vi "TEST.vi"() -> ()   [LabVIEW 2018, in "Config Parser BML.lvlib" / "Config Parser BML.lvclass"]
uses:
  Config Parser BML.lvclass
  Ctls/FRM Data - BML.ctl
  Ctls/OM - BML.ctl
  Ctls/Burst Length.ctl
  Ctls/RW Options.ctl
  Interfaces/File Parser Interface.lvlibp/Ctls/Protocol Type.ctl
  Interfaces/File Parser Interface.lvlibp/Interfaces/File Parser Interface/File Parser Interface.lvclass
  Interfaces/File Parser Interface.lvlibp
  C:/P4 Workspace/PC Client/Solutions/5g_eap/trunk/1.0/HiSi5GmmWave/Pattern_Gen_Tool/Interfaces/File Parser Interface.lvlibp/Interfaces/File Parser Interface/File Parser Interface.lvclass
panel:
  out "Array":T1[](array[typedef]) {"ChipID" format="%x"; "Start_Addr" format="%x"; "Data" format="%x"}
  out "error out":errorcluster
  in  "Config File":path
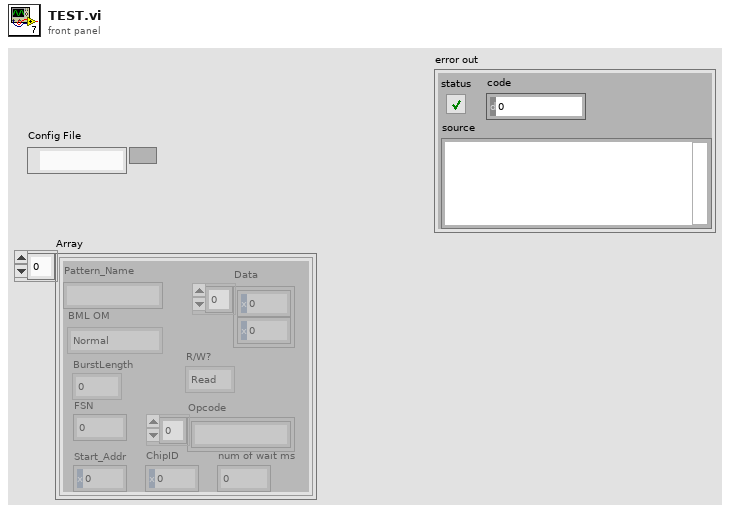
[diagram p1: front panel]
types:
  T1 = typedef "FRM Data - BML.ctl" = cluster{"Pattern_Name":string, "Data":u8[], "Start_Addr":u16, "ChipID":u8, "num of wait ms":i8, "Opcode":string[], "BML OM":T2, "BurstLength":T3, "FSN":u8, "R/W?":T4}
  T2 = typedef "OM - BML.ctl" = enum16{"Normal", "ImmeEffect", "InitSlaveID", "LoadData"}
  T3 = typedef "Burst Length.ctl" = enum8{"0", "2", "3", "4", "5", "8", "16", "32"}
  T4 = typedef "RW Options.ctl" = enum16{"Read", "Write", "R/W"}
  T5 = typedef "File Parser Interface.lvlibp/Protocol Type.ctl" = enum16{"BML_LS", "BML_HS", "SPI_3W", "SPI_4W"}
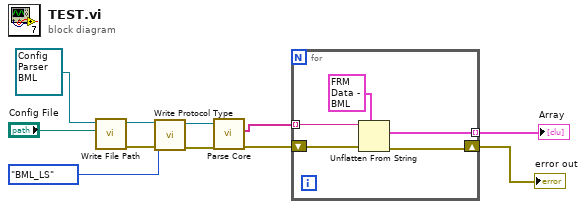
[diagram p0: block diagram]
diagram:
  n1 = call "Write File Path.vi"("File Path"="Config File", "File Parser Interface in"=refnum<class "Config Parser BML.lvclass"> refnum ("Config Parser BML.lvlib:Config Parser BML.lvclass")) -> ("error out"=w3:errorcluster, "File Parser Interface out"=w5:refnum<class "Config Parser BML.lvclass">)  [unwired: 8 in]
  n2 = call "Write Protocol Type.vi"("error in (no error)"=w3, "Protocol Type"=Protocol_Type."BML_LS", "File Parser Interface in"=w5) -> ("error out"=w2:errorcluster, "File Parser Interface out"=w4:refnum<class "Config Parser BML.lvclass">)  [unwired: 7 in]
  n3 = call-dynamic "Parse Core.vi"("error in (no error)"=w2, "Config Parser BML in"=w4) -> ("error out"=w7:errorcluster, "Config Array"=w6:string[])  [unwired: 7 in, 1 out]
  n4 = for {
    tunnel: [w15] -> w10 mode=indexing
    shift-right: [w13] -> w11
    shift-left: w7 -> [w14]
    tunnel: w6 -> [w12] mode=indexing
    n5 = Unflatten From String(type=T1 {"Pattern_Name"="", "Data"=[], "Start_Addr"=0, "ChipID"=1, "num of wait ms"=0, "Opcode"=[], "BML OM"=enum."Normal", "BurstLength"=enum."0", "FSN"=0, "R/W?"=enum."Read"} ("Frame Data"), binary string=w12, error in (no error)=w14) -> (value=w15:T1, error out=w13:errorcluster)  [unwired: 2 in, 1 out]
  }
  "error out" <- w11
  "Array" <- w10
